vi "MALT160T get several output.vi"() -> ()   [LabVIEW 2018]
uses:
  <instrlib>/AltonTech MALT/AltonTech MALT200817.lvlib
panel:
  in  "Block":i32
  out "Status":u8[](array[numeric]) format="%02x"
  in  "Address":i32=3 format="%02x"
  in  "stop":bool
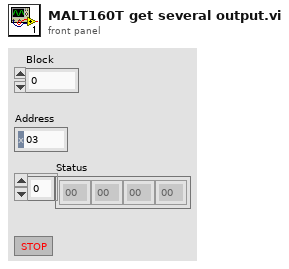
[diagram p1: front panel]
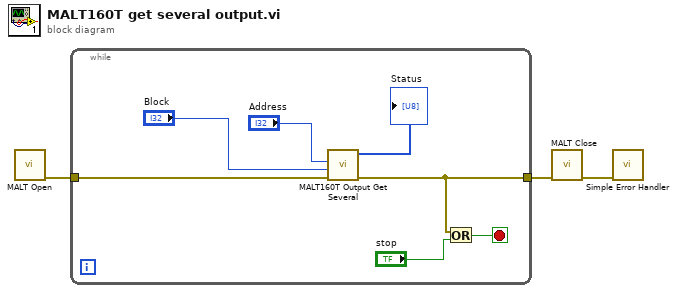
[diagram p0: block diagram]
diagram:
  n1 = call <instrlib>:"MALT Open.vi"() -> ("error out"=w3:errorcluster)  [unwired: 10 in, 1 out]
  n2 = while {
    tunnel: w3 -> [w10]
    tunnel: [w7] -> w2
    stop <- w5 stop-if-true
    n3 = call <instrlib>:"MALT160T Output Get Several.vi"("error in"=w10, "Block"="Block", "Address"="Address") -> ("error out"=w7:errorcluster, "Status"=→"Status":u8[])  [unwired: 7 in]
    n4 = Or(x=w7, y="stop") -> (x .or. y?=w5:bool)
  }
  n5 = call <instrlib>:"MALT Close.vi"("error in"=w2) -> ("error out"=w1:errorcluster)  [unwired: 10 in]
  n6 = call <vilib>:"Simple Error Handler.vi"("error in (no error)"=w1) -> ()  [unwired: 4 in, 5 out]
